vi "New Entity Template.vi"() -> (2 "New Entity Template":path)   [LabVIEW 2020, in "Conditum-Tools.lvlib"]
uses:
  Conditum-Tools.lvlib
  <vilib>/IlluminatedG/IG Conditum Base/Conditum/Conditum.lvlib
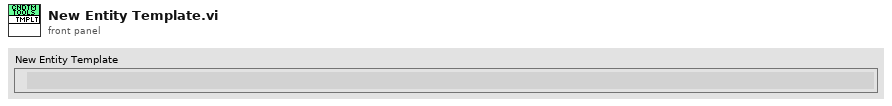
[diagram p1: front panel]
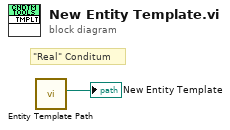
[diagram p0: block diagram]
diagram:
  # "\"Real\" Conditum"
  n1 = call <vilib>:"Entity Template Path.vi"() -> ("New Entity Template"=→"New Entity Template":path)  [unwired: 11 in]
